vi "Continuous Inverse CDF.vi"   [LabVIEW 2017, in "NI_Gmath.lvlib"]
doc: "Computes the continuous inverse cumulative distribution function (CDF) of the various distributions. You must manually select the polymorphic instance to use."
uses:
  <vilib>/gmath/NI_Gmath.lvlib
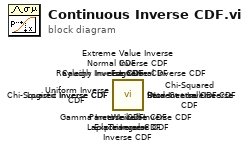
[diagram p0: block diagram]
diagram:
  n1 = call <vilib>:"Pareto Inverse CDF.vi"() -> ()  [unwired: 10 in, 2 out]
  n2 = call <vilib>:"Lognormal Inverse CDF.vi"() -> ()  [unwired: 10 in, 2 out]
  n3 = call <vilib>:"Logistic Inverse CDF.vi"() -> ()  [unwired: 10 in, 2 out]
  n4 = call <vilib>:"Chi-Squared (Non-Central) Inverse CDF.vi"() -> ()  [unwired: 10 in, 2 out]
  n5 = call <vilib>:"Laplace Inverse CDF.vi"() -> ()  [unwired: 10 in, 2 out]
  n6 = call <vilib>:"Extreme Value Inverse CDF.vi"() -> ()  [unwired: 10 in, 2 out]
  n7 = call <vilib>:"Rayleigh Inverse CDF.vi"() -> ()  [unwired: 10 in, 2 out]
  n8 = call <vilib>:"Weibull Inverse CDF.vi"() -> ()  [unwired: 10 in, 2 out]
  n9 = call <vilib>:"Uniform Inverse CDF.vi"() -> ()  [unwired: 10 in, 2 out]
  n10 = call <vilib>:"Triangular Inverse CDF.vi"() -> ()  [unwired: 10 in, 2 out]
  n11 = call <vilib>:"Student t Inverse CDF.vi"() -> ()  [unwired: 10 in, 2 out]
  n12 = call <vilib>:"Normal Inverse CDF.vi"() -> ()  [unwired: 10 in, 2 out]
  n13 = call <vilib>:"Gamma Inverse CDF.vi"() -> ()  [unwired: 10 in, 2 out]
  n14 = call <vilib>:"F Inverse CDF.vi"() -> ()  [unwired: 10 in, 2 out]
  n15 = call <vilib>:"Exp Inverse CDF.vi"() -> ()  [unwired: 10 in, 2 out]
  n16 = call <vilib>:"Chi-Squared Inverse CDF.vi"() -> ()  [unwired: 10 in, 2 out]
  n17 = call <vilib>:"Cauchy Inverse CDF.vi"() -> ()  [unwired: 10 in, 2 out]
  n18 = call <vilib>:"Beta Inverse CDF.vi"() -> ()  [unwired: 10 in, 2 out]
